vi "Reset Supply.vi"(8 "error in":errorcluster, 11 "PowerSupply in":refnum<class "PowerSupply.lvclass">) -> (0 "error out":errorcluster, 3 "PowerSupply out":refnum<class "PowerSupply.lvclass">)   [LabVIEW 2019, in "PowerSupply.lvlib" / "PowerSupply.lvclass"]
uses:
  Library/PowerSupply.lvclass
  Library/PowerSupply.lvclass/PowerSupply.ctl
  Custom Controls/Settings.ctl
  Custom Controls/Sense Point.ctl
  Custom Controls/OCP Mode.ctl
  builds/Engine/Engine.lvlibp/Project/Engine.lvclass
  builds/Instruments/Instruments.lvlibp/Library/Instruments.lvclass
  builds/Instruments/Instruments.lvlibp/Private/Polymorphic/Special/Event from String.vi
  builds/Instruments/Instruments.lvlibp
  C:/Users/Public/Documents/Development/builds/Instruments/Instruments.lvlibp/Library/Instruments.lvclass
  C:/Users/Public/Documents/Development/builds/Tools/Config.lvlibp/Config.lvclass
  C:/Users/Public/Documents/Development/builds/Engine/Engine.lvlibp/Project/Engine.lvclass
  C:/Users/Public/Documents/Development/builds/Engine/Panel Manager.lvlibp/Panel Actor/Panel Actor.lvclass
  C:/Users/Public/Documents/Development/builds/Engine/Monitored Actor.lvlibp/Monitored Actor/Monitored Actor/Monitored Actor.lvclass
  C:/Users/Public/Documents/Development/builds/Engine/Actor Framework.lvlibp/1abvi3w/vi.lib/ActorFramework/Actor/Actor.lvclass
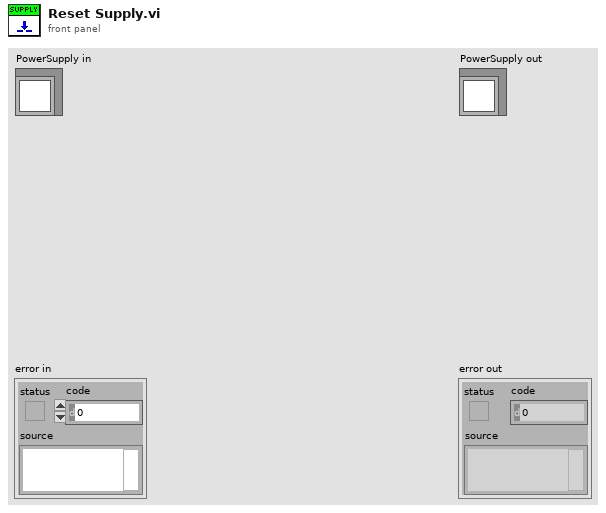
[diagram p1: front panel]
types:
  T1 = typedef "PowerSupply.lvlib/PowerSupply.lvclass/Settings.ctl" = cluster{"Voltage":dbl, "Current":dbl, "Output":bool, "OverVolt_Protect":dbl, "OverCurrent_Protect":dbl, "OVP":bool, "OCP":bool, "Interlock":bool, "Volt_Ramp":dbl, "Current_Ramp":dbl, "Sense Point":T2, "OCP Mode":T3, "Sharing":bool}
  T2 = typedef "PowerSupply.lvlib/PowerSupply.lvclass/Sense Point.ctl" = enum16{"Local", "Remote"}
  T3 = typedef "PowerSupply.lvlib/PowerSupply.lvclass/OCP Mode.ctl" = enum16{"Shutdown", "Foldback"}
  T4 = cluster{"Timestamp":timestamp, "Description":string, "Data":string}
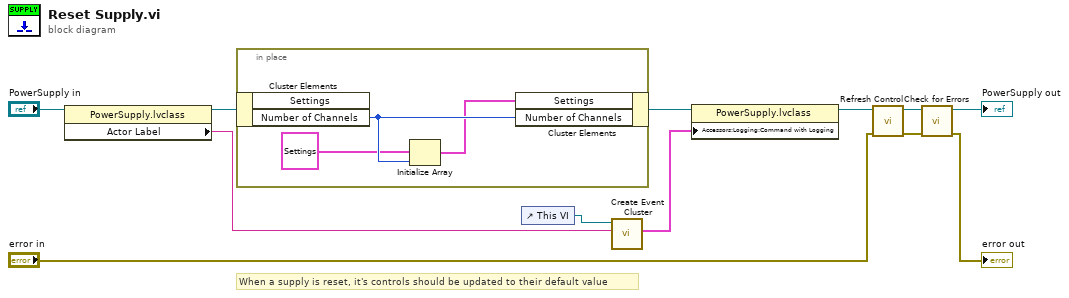
[diagram p0: block diagram]
diagram:
  # "When a supply is reset, it's controls should be updated to their default value"
  n1 = property class="PowerSupply.lvclass"(reference="PowerSupply in") -> (reference out=w3:refnum<class "PowerSupply.lvclass">, "Actor Label"=w2:string)  [unwired: 1 in, 1 out]
  n2 = in-place {
    n3 = in-place-cluster #1(w3) -> ("Number of Channels"=w15:i32)  [unwired: 1 out]
    n4 = Initialize Array(T1 {"Voltage"=0.0, "Current"=0.0, "Output"=FALSE, "OverVolt_Protect"=0.0, "OverCurrent_Protect"=0.0, "OVP"=FALSE, "OCP"=FALSE, "Interlock"=FALSE, "Volt_Ramp"=0.0, "Current_Ramp"=0.0, "Sense Point"=enum."Local", "OCP Mode"=enum."Shutdown", "Sharing"=FALSE} ("Settings"), w15) -> (w13:T1[])
    n5 = in-place-cluster #1("Settings"=w13, "Number of Channels"=w15) -> (w7:refnum<class "PowerSupply.lvclass">)
  }
  n6 = control-ref of="This VI"() -> (w5:refnum<vi>)
  n7 = call-poly "Create Event Cluster.vi"("Value"=w2, "VI Refnum"=w5) -> ("Event Data"=w1:T4)  [unwired: 9 in]
  n8 = property class="PowerSupply.lvclass"(reference=w7, "Accessors:Logging:Command with Logging"=w1) -> (reference out=w6:refnum<class "PowerSupply.lvclass">)  [unwired: 1 in, 1 out]
  n9 = call "Refresh Control.vi"("error in"="error in", "PowerSupply in"=w6) -> ("error out"=w10:errorcluster, "PowerSupply out"=w11:refnum<class "PowerSupply.lvclass">)  [unwired: 8 in]
  n10 = call "Check for Errors.vi"("error in"=w10, "Engine in"=w11) -> ("error out"=→"error out":errorcluster, "Engine out"=→"PowerSupply out":refnum<class "PowerSupply.lvclass">)  [unwired: 8 in]
